vi "SSC Digital Frequency Counter Measure Frequency.vi"(0 "Digital SSC in":T1[](array[typedef]), 11 "error in":errorcluster) -> (4 "Digital SSC out":T1[](array[typedef]), 6 "Per-Instrument Frequencies (Hz)":dbl[][](array[numeric]), 15 "error out":errorcluster)   [LabVIEW 2020]
doc: "Measures the frequency on the specified pin(s) and pin group(s) over the configured measurement time."
uses:
  SSC Digital.ctl
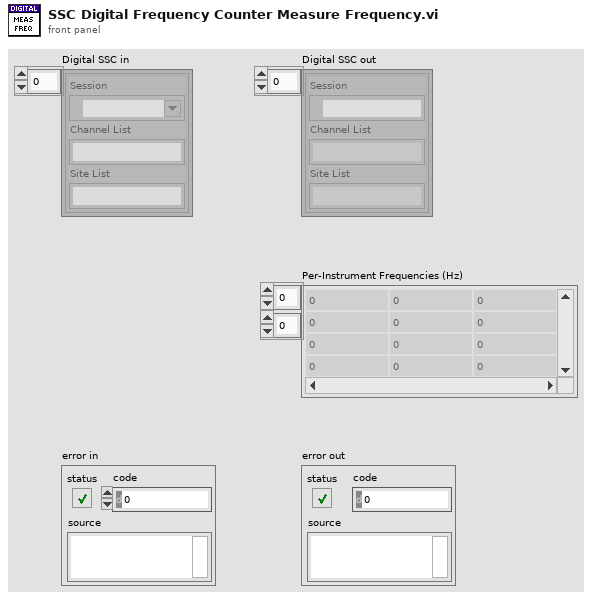
[diagram p1: front panel]
types:
  T1 = typedef "SSC Digital.ctl" = cluster{"Session":refnum<k15>, "Channel List":string, "Site List":string}
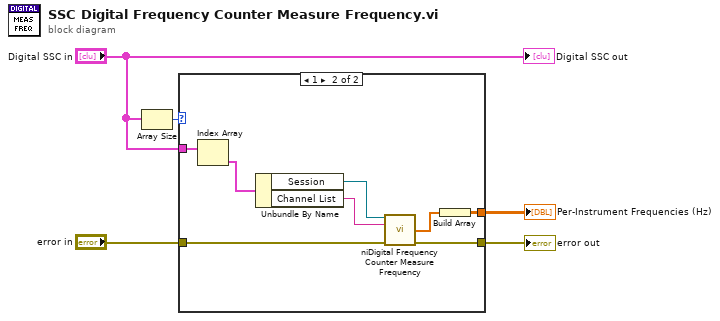
[diagram p0: block diagram]
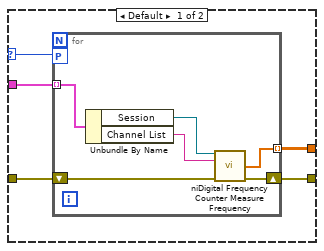
[diagram p2: hidden frame]
diagram:
  n1 = Array Size(array="Digital SSC in") -> (size(s)=w2:i32)
  n2 = case shown="1" w2 {
    selector: w2 -> [w7 _]
    tunnel: "error in" -> [w10 w24]
    tunnel: [w9 w17] -> w4
    tunnel: [w8 w22] -> w3
    tunnel: "Digital SSC in" -> [w6 w21]
    frame Default {
      n3 = for {
        tunnel: w6 -> [w15] mode=indexing
        tunnel: [w16] -> w9 mode=indexing
        workers-P: w7 -> [_]
        shift-right: [w12] -> w8
        shift-left: w10 -> [w13]
        n4 = Unbundle By Name(w15) -> ("Session"=w14:refnum<k15>, "Channel List"=w11:string)
        n5 = call <instrlib>:"niDigital Frequency Counter Measure Frequency.vi"("instrument handle"=w14, "channel list"=w11, "error in"=w13) -> ("frequencies (Hz)"=w16:dbl[], "error out"=w12:errorcluster)  [unwired: 10 in, 1 out]
      }
    }
    frame 1 {
      n6 = Index Array(array=w21) -> (element=w18:T1)  [unwired: 1 in]
      n7 = Unbundle By Name(w18) -> ("Session"=w20:refnum<k15>, "Channel List"=w19:string)
      n8 = call <instrlib>:"niDigital Frequency Counter Measure Frequency.vi"("instrument handle"=w20, "channel list"=w19, "error in"=w24) -> ("frequencies (Hz)"=w23:dbl[], "error out"=w22:errorcluster)  [unwired: 10 in, 1 out]
      n9 = Build Array(w23) -> (w17:dbl[][])
    }
  }
  "error out" <- w3
  "Per-Instrument Frequencies (Hz)" <- w4
  "Digital SSC out" <- "Digital SSC in"
